vi "Init.vi"(8 "error in (no error)":errorcluster, 10 "Colour":u32(colorbox), 11 "GameEl in":refnum<class "GameEl.lvclass">) -> (0 "error out":errorcluster, 3 "GameEl out":refnum<class "GameEl.lvclass">)   [LabVIEW 2021, in "GameEl.lvclass"]
uses:
  GameEl.lvclass
  GameEl.lvclass/GameEl.ctl
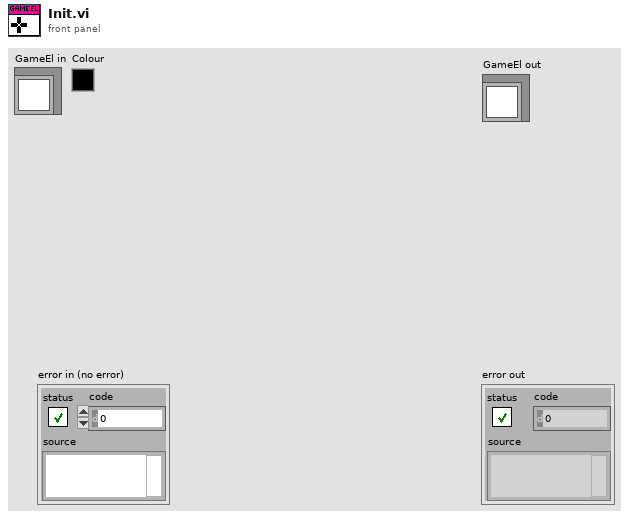
[diagram p1: front panel]
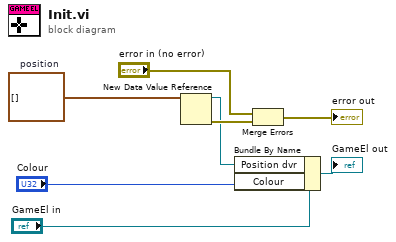
[diagram p0: block diagram]
diagram:
  w2 = cluster{"x":dbl, "y":dbl}[] []  # position
  n1 = New Data Value Reference(data value=w2) -> (data value reference=w3:refnum<data-value>, error out=w5:errorcluster)  [unwired: 1 in]
  n2 = Bundle By Name(cluster="GameEl in", "Position dvr"=w3, "Colour"="Colour") -> (→"GameEl out":refnum<class "GameEl.lvclass">)
  n3 = Merge Errors("error in (no error)", w5) -> (→"error out":errorcluster)
